vi "PCO_GetGeneral.vi"() -> ()   [LabVIEW 2011]
uses:
  SC2_Cam64.dll
panel:
  out "PCO_FW_Vers":T1(array[cluster])
  out "PCO_HW_Vers":T2(array[cluster])
  out "PCO_CameraType":T3={"wCamType"=137363456, "wCamSubType"=33940, "dummy"=1966081, "dwSerialNumber"=32928, "dwHWVersion"=131073, "dwFWVersion"=0, "wInterfaceType"=0}
  out "PCO_general":T4={"dwCamHealthWarnings"=0, "dwCamHealthErrors 2"=0, "dwCamHealthStatus 3"=393216, "sCCDTemperature"=308, "sCamTemperature 2"=30, "sPowerSupplyTemperature 3"=24}
  out "PCO_camertype":u16[](array[numeric])=[1364, 2096, 0, 0, 33940, 30, 1, 0, 32928, 2, 1, 3, 21576, 19779, 18753, 78, 0, 0, 0, 0, 1, 3, 12, 0, 0, 0, 0, 0, 0, 0, 0, 0, 0, 0, 0, 0, 0, 0, 0, 0, 0, 0, 0, 21576, 20547, 22351, 21061, 0, 0, 0, 0, 1, 3, 12, 0, 0, 0, 0, 0, 0, 0, 0, 0, 0, 0, 0, 0, 0, 0, 0, 0, 0, 0, 0, 21576, 16707, 16964, 17490, 0, 0, 0, 0, 60676, 0, 4260, 0, 0, 0, 0, 0, 0, 0, 0, 0, 0, 0, 0, 0, 0, 0, 0, 0, 0, 0, 0, 0, 0, 0, 0, 0, 0, 0, 0, 0, 0, 0, 0, 0, 0, 0, 0, 0, 0, 0, 0, 0, 0, 0, 0, 0, 0, 0, 0, 0, 0, 0, 0, 0, 0, 0, 0, 0, 0, 0, 0, 0, 0, 0, 0, 0, 0, 0, 0, 0, 0, 0, 0, 0, 0, 0, 0, 0, 0, 0, 0, 0, 0, 0, 0, 0, 0, 0, 0, 0, 0, 0, 0, 0, 0, 0, 0, 0, 0, 0, 0, 0, 0, 0, 0, 0, 0, 0, 0, 0, 0, 0, 0, 0, 0, 0, 0, 0, 0, 0, 0, 0, 0, 0, 0, 0, 0, 0, 0, 0, 0, 0, 0, 0, 0, 0, 0, 0, 0, 0, 0, 0, 0, 0, 0, 0, 0, 0, 0, 0, 0, 0, 0, 0, 0, 0, 0, 0, 0, 0, 0, 0, 0, 0, 0, 0, 0, 0, 0, 0, 0, 0, 0, 0, 0, 0, 0, 0, 0, 0, 0, 0, 0, 0, 0, 0, 0, 0, 0, 0, 0, 0, 0, 0, 0, 0, 0, 0, 0, 0, 0, 0, 0, 0, 0, 0, 0, 0, 0, 0, 0, 0, 0, 0, 0, 0, 0, 0, 0, 0, 0, 0, 0, 0, 0, 0, 0, 0, 0, 0, 0, 0, 0, 0, 0, 0, 0, 0, 4, 24909, 28265, 29984, 80, 0, 0, 0, 0, 544, 12, 0, 0, 0, 0, 0, 0, 0, 0, 0, 0, 0, 0, 0, 0, 0, 0, 0, 0, 0, 0, 0, 0, 24909, 28265, 17952, 18256, 65, 0, 0, 0, 544, 12, 0, 0, 0, 0, 0, 0, 0, 0, 0, 0, 0, 0, 0, 0, 0, 0, 0, 0, 0, 0, 0, 0, 25928, 25697, 17184, 19536, 68, 0, 0, 0, 0, 0, 0, 0, 0, 0, 0, 0, 0, 0, 0, 0, 0, 0, 0, 0, 0, 0, 0, 0, 0, 0, 0, 0, 24909, 28265, 16928, 28527, 27764, 24943, 25956, 114, 7, 1, 0, 0, 0, 0, 0, 0, 0, 0, 0, 0, 0, 0, 0, 0, 0, 0, 0, 0, 0, 0, 0, 0, 0, 0, 0, 0, 0, 0, 0, 0, 0, 0, 0, 0, 0, 0, 0, 0, 0, 0, 0, 0, 0, 0, 0, 0, 0, 0, 0, 0, 0, 0, 0, 0, 0, 0, 0, 0, 0, 0, 0, 0, 0, 0, 0, 0, 0, 0, 0, 0, 0, 0, 0, 0, 0, 0, 0, 0, 0, 0, 0, 0, 0, 0, 0, 0, 0, 0, 0, 0, 0, 0, 0, 0, 0, 0, 0, 0, 0, 0, 0, 0, 0, 0, 0, 0, 0, 0, 0, 0, 0, 0, 0, 0, 0, 0, 0, 0, 0, 0, 0, 0, 0, 0, 0, 0, 0, 0, 0, 0, 0, 0, 0, 0, 0, 0, 0, 0, 0, 0, 0, 0, 0, 0, 0, 0, 0, 0, 0, 0, 0, 0, 0, 0, 0, 0, 0, 0, 0, 0, 0, 0, 0, 0, 0, 0, 0, 0, 0, 0, 0, 0, 0, 0, 0, 0, 0, 0, 0, 0, 0, 0, 0, 0, 0, 0, 0, 0, 0, 0, 0, 0, 0, 0, 0, 0, 0, 0, 0, 0, 0, 0, 0, 0, 0, 0, 0, 0, 0, 0, 0, 0, 0, 0, 61176, 3568, 0, 0, 0, 0, 0, 0, 0, 0, 0, 0, 0, 0, 0, 0, 0, 0, 0, 0, 0, 0, 0, 0, 0, 0, 0, 0, 0, 0, 0, 0, 0, 0, 0, 0, 0, 0, 0]
  out "wPCO_general":u16[](array[numeric])=[1460, 1460, 1364, 2096, 0, 0, 33940, 30, 1, 0, 32928, 2, 1, 3, 21576, 19779, 18753, 78, 0, 0, 0, 0, 1, 3, 12, 0, 0, 0, 0, 0, 0, 0, 0, 0, 0, 0, 0, 0, 0, 0, 0, 0, 0, 0, 0, 21576, 20547, 22351, 21061, 0, 0, 0, 0, 1, 3, 12, 0, 0, 0, 0, 0, 0, 0, 0, 0, 0, 0, 0, 0, 0, 0, 0, 0, 0, 0, 0, 21576, 16707, 16964, 17490, 0, 0, 0, 0, 60676, 0, 4260, 0, 0, 0, 0, 0, 0, 0, 0, 0, 0, 0, 0, 0, 0, 0, 0, 0, 0, 0, 0, 0, 0, 0, 0, 0, 0, 0, 0, 0, 0, 0, 0, 0, 0, 0, 0, 0, 0, 0, 0, 0, 0, 0, 0, 0, 0, 0, 0, 0, 0, 0, 0, 0, 0, 0, 0, 0, 0, 0, 0, 0, 0, 0, 0, 0, 0, 0, 0, 0, 0, 0, 0, 0, 0, 0, 0, 0, 0, 0, 0, 0, 0, 0, 0, 0, 0, 0, 0, 0, 0, 0, 0, 0, 0, 0, 0, 0, 0, 0, 0, 0, 0, 0, 0, 0, 0, 0, 0, 0, 0, 0, 0, 0, 0, 0, 0, 0, 0, 0, 0, 0, 0, 0, 0, 0, 0, 0, 0, 0, 0, 0, 0, 0, 0, 0, 0, 0, 0, 0, 0, 0, 0, 0, 0, 0, 0, 0, 0, 0, 0, 0, 0, 0, 0, 0, 0, 0, 0, 0, 0, 0, 0, 0, 0, 0, 0, 0, 0, 0, 0, 0, 0, 0, 0, 0, 0, 0, 0, 0, 0, 0, 0, 0, 0, 0, 0, 0, 0, 0, 0, 0, 0, 0, 0, 0, 0, 0, 0, 0, 0, 0, 0, 0, 0, 0, 0, 0, 0, 0, 0, 0, 0, 0, 0, 0, 0, 0, 0, 0, 0, 0, 0, 0, 0, 0, 0, 0, 0, 0, 0, 0, 0, 0, 0, 0, 0, 0, 4, 24909, 28265, 29984, 80, 0, 0, 0, 0, 544, 12, 0, 0, 0, 0, 0, 0, 0, 0, 0, 0, 0, 0, 0, 0, 0, 0, 0, 0, 0, 0, 0, 0, 24909, 28265, 17952, 18256, 65, 0, 0, 0, 544, 12, 0, 0, 0, 0, 0, 0, 0, 0, 0, 0, 0, 0, 0, 0, 0, 0, 0, 0, 0, 0, 0, 0, 25928, 25697, 17184, 19536, 68, 0, 0, 0, 0, 0, 0, 0, 0, 0, 0, 0, 0, 0, 0, 0, 0, 0, 0, 0, 0, 0, 0, 0, 0, 0, 0, 0, 24909, 28265, 16928, 28527, 27764, 24943, 25956, 114, 7, 1, 0, 0, 0, 0, 0, 0, 0, 0, 0, 0, 0, 0, 0, 0, 0, 0, 0, 0, 0, 0, 0, 0, 0, 0, 0, 0, 0, 0, 0, 0, 0, 0, 0, 0, 0, 0, 0, 0, 0, 0, 0, 0, 0, 0, 0, 0, 0, 0, 0, 0, 0, 0, 0, 0, 0, 0, 0, 0, 0, 0, 0, 0, 0, 0, 0, 0, 0, 0, 0, 0, 0, 0, 0, 0, 0, 0, 0, 0, 0, 0, 0, 0, 0, 0, 0, 0, 0, 0, 0, 0, 0, 0, 0, 0, 0, 0, 0, 0, 0, 0, 0, 0, 0, 0, 0, 0, 0, 0, 0, 0, 0, 0, 0, 0, 0, 0, 0, 0, 0, 0, 0, 0, 0, 0, 0, 0, 0, 0, 0, 0, 0, 0, 0, 0, 0, 0, 0, 0, 0, 0, 0, 0, 0, 0, 0, 0, 0, 0, 0, 0, 0, 0, 0, 0, 0, 0, 0, 0, 0, 0, 0, 0, 0, 0, 0, 0, 0, 0, 0, 0, 0, 0, 0, 0, 0, 0, 0, 0, 0, 0, 0, 0, 0, 0, 0, 0, 0, 0, 0, 0, 0, 0, 0, 0, 0, 0, 0, 0, 0, 0, 0, 0, 0, 0, 0, 0, 0, 0, 0, 0, 0, 0, 0, 0, 61176, 3568, 0, 0, 0, 0, 0, 0, 0, 0, 0, 0, 0, 0, 0, 0, 0, 0, 0, 0, 0, 0, 0, 0, 0, 0, 0, 0, 0, 0, 0, 0, 0, 0, 0, 0, 0, 0, 0, 0, 0, 0, 0, 6, 0, 308, 30, 24, 0, 0, 0, 0, 0, 0, 0, 0, 0, 0, 0, 0, 0, 0, 0, 0, 0, 0, 0, 0, 0, 0, 0, 0, 0, 0, 0, 0, 0, 0, 0, 0, 0, 0, 0, 0, 0]
  out "error out":errorcluster
  in  "error in (no error)":errorcluster
  out "return type":u32 format="%x"
  out "Handle Out":u64=176713696
  in  "Handle":u64=176713696
  # "2148151298:empty string,\n#define PCO_ERROR_SDKDLL_NESTEDBUFFERSIZE           0x80003001 // The wSize of an embedded buffer is to small.\n#define PCO_ERROR_SDKDLL_BUFFERSIZE                 0x80003002 // The wSize of a buffer is to small."
  # "typedef struct\n{\n  WORD        wSize;                   // Sizeof this struct\n  WORD        ZZwAlignDummy1;\n  PCO_CameraType strCamType;       1364    // previous described structure // 1368\n  DWORD       dwCamHealthWarnings;     // Warnings in camera system\n  DWORD       dwCamHealthErrors;       // Errors in camera system\n  DWORD       dwCamHealthStatus;       // Status of camera system      // 1380\n  SHORT       sCCDTemperature;         // CCD temperature\n  SHORT       sCamTemperature;         // Camera temperature           // 1384\n  SHORT       sPowerSupplyTemperature; // Power device temperature\n  WORD        ZZwDummy[37];                                            // 1460\n} PCO_General;"
  # "typedef struct\n{\n  WORD        wSize;                   // Sizeof this struct\n  WORD        wCamType;                // Camera type\n  WORD        wCamSubType;             // Camera sub type\n  WORD        ZZwAlignDummy1;\n  DWORD       dwSerialNumber;          // Serial number of camera // 12\n  DWORD       dwHWVersion;             // Hardware version number\n  DWORD       dwFWVersion;             // Firmware version number\n  WORD        wInterfaceType;          // Interface type          // 22\n  PCO_HW_Vers strHardwareVersion;      // Hardware versions of all boards // 644\n  PCO_FW_Vers strFirmwareVersion;      // Firmware versions of all devices // 1286\n  WORD        ZZwDummy[39];                                       // 1364\n} PCO_CameraType;"
  # "typedef struct\n{\n  WORD                   BoardNum;       // number of devices\n  PCO_SC2_Hardware_DESC  Board[PCO_MAXVERSIONHW];// 622\n}\nPCO_HW_Vers;\n\ntypedef struct\n{\n  WORD                   DeviceNum;       // number of devices\n  PCO_SC2_Firmware_DESC  Device[PCO_MAXVERSIONFW];// 642\n}\nPCO_FW_Vers;"
  # "typedef struct\n{\n  char  szName[16];      // string with board name\n  WORD  wBatchNo;        // production batch no\n  WORD  wRevision;       // use range 0 to 99\n  WORD  wVariant;        // variant    // 22\n  WORD  ZZwDummy[20];    //            // 62\n}\nPCO_SC2_Hardware_DESC;\n\ntypedef struct\n{\n  char  szName[16];      // string with device name\n  BYTE  bMinorRev;       // use range 0 to 99\n  BYTE  bMajorRev;       // use range 0 to 255\n  WORD  wVariant;        // variant    // 20\n  WORD  ZZwDummy[22];    //            // 64\n}\nPCO_SC2_Firmware_DESC;"
  # "#define PCO_MAXVERSIONHW   10\n#define PCO_MAXVERSIONFW   10"
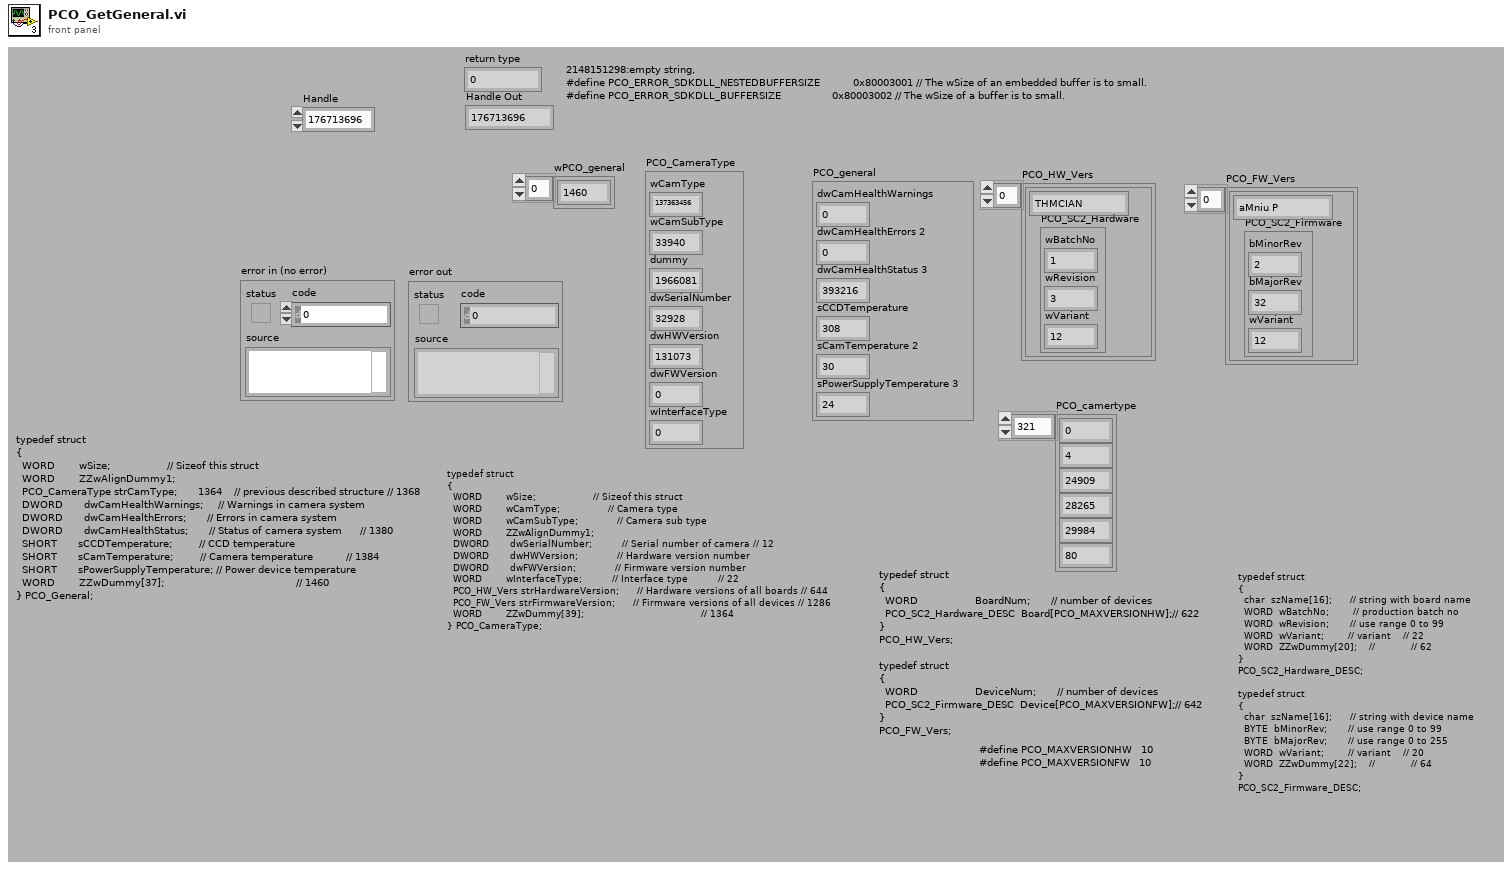
[diagram p1: front panel]
types:
  T1 = cluster{string, "PCO_SC2_Firmware":cluster{"bMinorRev":u8, "bMajorRev":u8, "wVariant":u16}}[]
  T2 = cluster{string, "PCO_SC2_Hardware":cluster{"wBatchNo":u16, "wRevision":u16, "wVariant":u16}}[]
  T3 = cluster{"wCamType":i32, "wCamSubType":i32, "dummy":i32, "dwSerialNumber":i32, "dwHWVersion":i32, "dwFWVersion":i32, "wInterfaceType":i32}
  T4 = cluster{"dwCamHealthWarnings":u32, "dwCamHealthErrors 2":u32, "dwCamHealthStatus 3":u32, "sCCDTemperature":i16, "sCamTemperature 2":i16, "sPowerSupplyTemperature 3":i16}
  T5 = cluster{"bMinorRev":u8, "bMajorRev":u8, "wVariant":u16}
  T6 = cluster{"wBatchNo":u16, "wRevision":u16, "wVariant":u16}
  T7 = cluster{string, "PCO_SC2_Hardware_DESC [62bytes]":cluster{"wBatchNo":u16, "wRevision":u16, "wVariant":u16}}
  T8 = cluster{string, "PCO_SC2_Firmware_DESC [64bytes]":cluster{"bMinorRev":u8, "bMajorRev":u8, "wVariant":u16}}
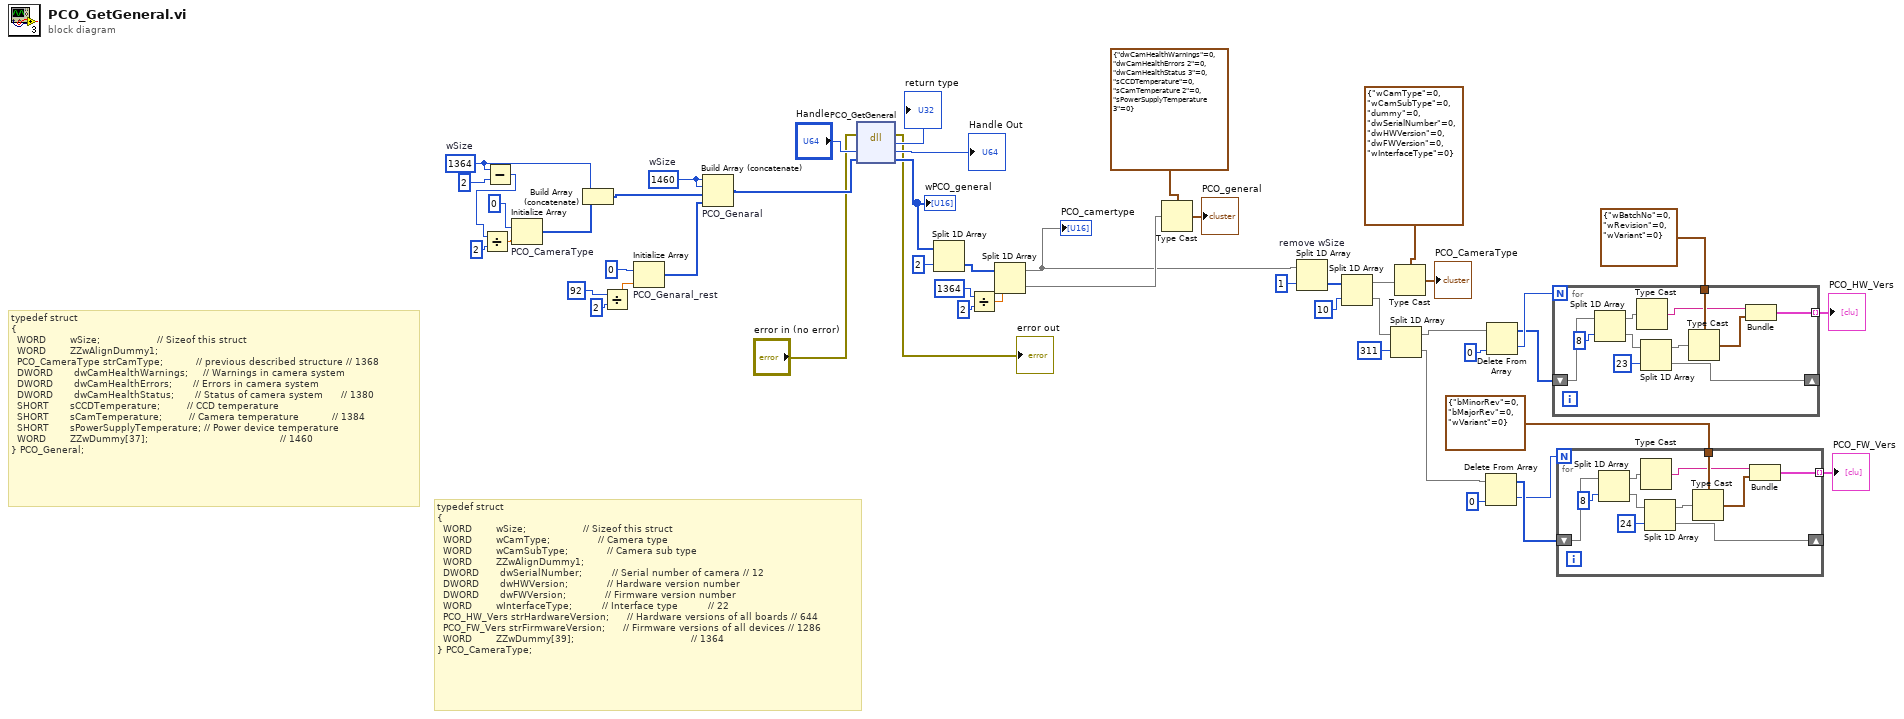
[diagram p0: block diagram]
diagram:
  w32 = u16 1364  # wSize
  w47 = u16 1460  # wSize
  # "typedef struct\n{\n  WORD        wSize;                   // Sizeof this struct\n  WORD        wCamType;                // Camera type\n  WORD        wCamSubType;             // Camera sub type\n  WORD        ZZwAlignDummy1;\n  DWORD       dwSerialNumber;          // Serial number of camera // 12\n  DWORD       dwHWVersion;             // Hardware version number\n  DWORD       dwFWVersion;             // Firmware version number\n  WORD        wInterfaceType;          // Interface type          // 22\n  PCO_HW_Vers strHardwareVersion;      // Hardware versions of all boards // 644\n  PCO_FW_Vers strFirmwareVersion;      // Firmware versions of all devices // 1286\n  WORD        ZZwDummy[39];                                       // 1364\n} PCO_CameraType;"
  # "typedef struct\n{\n  WORD        wSize;                   // Sizeof this struct\n  WORD        ZZwAlignDummy1;\n  PCO_CameraType strCamType;           // previous described structure // 1368\n  DWORD       dwCamHealthWarnings;     // Warnings in camera system\n  DWORD       dwCamHealthErrors;       // Errors in camera system\n  DWORD       dwCamHealthStatus;       // Status of camera system      // 1380\n  SHORT       sCCDTemperature;         // CCD temperature\n  SHORT       sCamTemperature;         // Camera temperature           // 1384\n  SHORT       sPowerSupplyTemperature; // Power device temperature\n  WORD        ZZwDummy[37];                                            // 1460\n} PCO_General;"
  n1 = Subtract(x=w32, y=2) -> (x-y=w30:i32)
  n2 = Divide(x=w30, y=u16 2) -> (x/y=w46:dbl)
  n3 = Initialize Array "PCO_CameraType"(u16 0 ("element"), w46) -> (w37:u16[])
  n4 = Build Array (concatenate)(w32, w37) -> (w36:u16[])
  n5 = Divide(x=92, y=u16 2) -> (x/y=w40:dbl)
  n6 = Initialize Array "PCO_Genaral_rest"(u16 0 ("element"), w40) -> (w43:u16[])
  n7 = Build Array (concatenate) "PCO_Genaral"(w47, w47, w36, w43) -> (w39:u16[])
  n8 = dll-call lib="C:/Program Files/colibri/Drivers/PCO.Camera/SC2_Cam*.*" fn="PCO_GetGeneral"(error in="error in (no error)", "Handle"="Handle", "PCO_general"=w39) -> (error out=→"error out":errorcluster, "return type"=→"return type":u32, "Handle"=→"Handle Out":u64, "PCO_general"=w35:u16[])  [unwired: 2 in, 1 out]
  "wPCO_general" <- w35
  n9 = Split 1D Array(array=w35, index=2) -> (second subarray=w33:u16[])  [unwired: 1 out]
  n10 = Divide(x=1364, y=u16 2) -> (x/y=w27:dbl)
  n11 = Split 1D Array(array=w33, index=w27) -> (first subarray=w23:u16[], second subarray=w25:u16[])
  "PCO_camertype" <- w23
  n12 = Type Cast(type=T4 {"dwCamHealthWarnings"=0, "dwCamHealthErrors 2"=0, "dwCamHealthStatus 3"=0, "sCCDTemperature"=0, "sCamTemperature 2"=0, "sPowerSupplyTemperature 3"=0}, x=w25) -> (*(type *) &x=→"PCO_general":T4)
  n13 = Split 1D Array "remove wSize"(array=w23, index=1) -> (second subarray=w21:u16[])  [unwired: 1 out]
  n14 = Split 1D Array(array=w21, index=10) -> (first subarray=w19:u16[], second subarray=w16:u16[])
  n15 = Split 1D Array(array=w16, index=311) -> (first subarray=w14:u16[], second subarray=w11:u16[])
  n16 = Type Cast(type=T3 {"wCamType"=0, "wCamSubType"=0, "dummy"=0, "dwSerialNumber"=0, "dwHWVersion"=0, "dwFWVersion"=0, "wInterfaceType"=0}, x=w19) -> (*(type *) &x=→"PCO_CameraType":T3)
  n17 = Delete From Array(array=w11, index=0) -> (deleted portion=w5:u16, array with subset deleted=w6:u16[])  [unwired: 1 in]
  n18 = Delete From Array(array=w14, index=0) -> (deleted portion=w10:u16, array with subset deleted=w9:u16[])  [unwired: 1 in]
  n19 = for {
    N: w10 -> [_]
    shift-right: [w56] -> _
    shift-left: w9 -> [w61]
    tunnel: T6 {"wBatchNo"=0, "wRevision"=0, "wVariant"=0} ("PCO_SC2_Hardware_DESC [62bytes]") -> [w54]
    tunnel: [w51] -> w7 mode=indexing
    n20 = Split 1D Array(array=w61, index=8) -> (first subarray=w59:u16[], second subarray=w58:u16[])
    n21 = Type Cast(x=w59) -> (*(type *) &x=w53:string)  [unwired: 1 out]
    n22 = Split 1D Array(array=w58, index=23) -> (first subarray=w55:u16[], second subarray=w56:u16[])
    n23 = Type Cast(type=w54, x=w55) -> (*(type *) &x=w52:T6)
    n24 = Bundle(w53, "PCO_SC2_Hardware_DESC [62bytes]"=w52) -> (w51:T7)  [unwired: 1 out]
  }
  "PCO_HW_Vers" <- w7
  n25 = for {
    N: w5 -> [_]
    shift-right: [w67] -> _
    shift-left: w6 -> [w72]
    tunnel: T5 {"bMinorRev"=0, "bMajorRev"=0, "wVariant"=0} ("PCO_SC2_Firmware_DESC [64bytes]") -> [w65]
    tunnel: [w62] -> w3 mode=indexing
    n26 = Split 1D Array(array=w72, index=8) -> (first subarray=w70:u16[], second subarray=w69:u16[])
    n27 = Type Cast(x=w70) -> (*(type *) &x=w64:string)  [unwired: 1 out]
    n28 = Split 1D Array(array=w69, index=24) -> (first subarray=w66:u16[], second subarray=w67:u16[])
    n29 = Type Cast(type=w65, x=w66) -> (*(type *) &x=w63:T5)
    n30 = Bundle(w64, "PCO_SC2_Firmware_DESC [64bytes]"=w63) -> (w62:T8)  [unwired: 1 out]
  }
  "PCO_FW_Vers" <- w3
